vi "Decorator1_Main.vi"() -> ()   [LabVIEW 2020]
doc: "Main VI to test the DecoratorPattern"
uses:
  Espresso_class/Espresso.lvclass
  C:/Projects/DesignPatterns/DecoratorPattern/Beverage_class/Beverage.lvclass
  DarkRost_class/DarkRost.lvclass
  HouseBlend_class/HouseBlend.lvclass
  Decaf_class/Decaf.lvclass
  Milk_class/Milk.lvclass
  Soy_class/Soy.lvclass
  Mocha_class/Mocha.lvclass
  Whip_class/Whip.lvclass
  Beverage_class/Beverage.lvclass
panel:
  in  "Whip":u16(ring) items=["None", "Single", "Double"]
  in  "Mocha":u16(ring) items=["None", "Single", "Double"]
  in  "Coffee type":T1(radio)
  in  "Milk type":enum32{"No Milk", "Normal Milk", "Soy Milk"}(radio)
  out "Description and cost":string
  # "This Application shows how the Decorator Pattern could be implelemted based on the book:\nFirst Design Patterns,  Eric Freeman et. al. 2004. O'Reilly Media, Inc.\nhttp://oreilly.com/catalog/hfdesignpat/chapter/ch03.pdf\nCheers,\nMike"
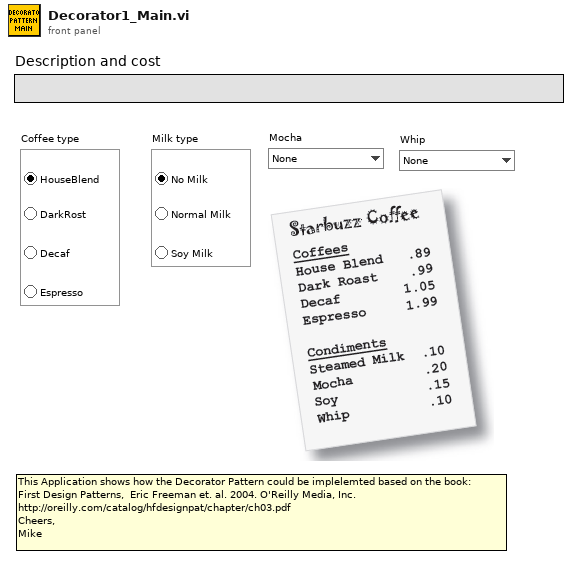
[diagram p1: front panel]
types:
  T1 = enum32{"HouseBlend", "DarkRost", "Decaf", "Espresso"}
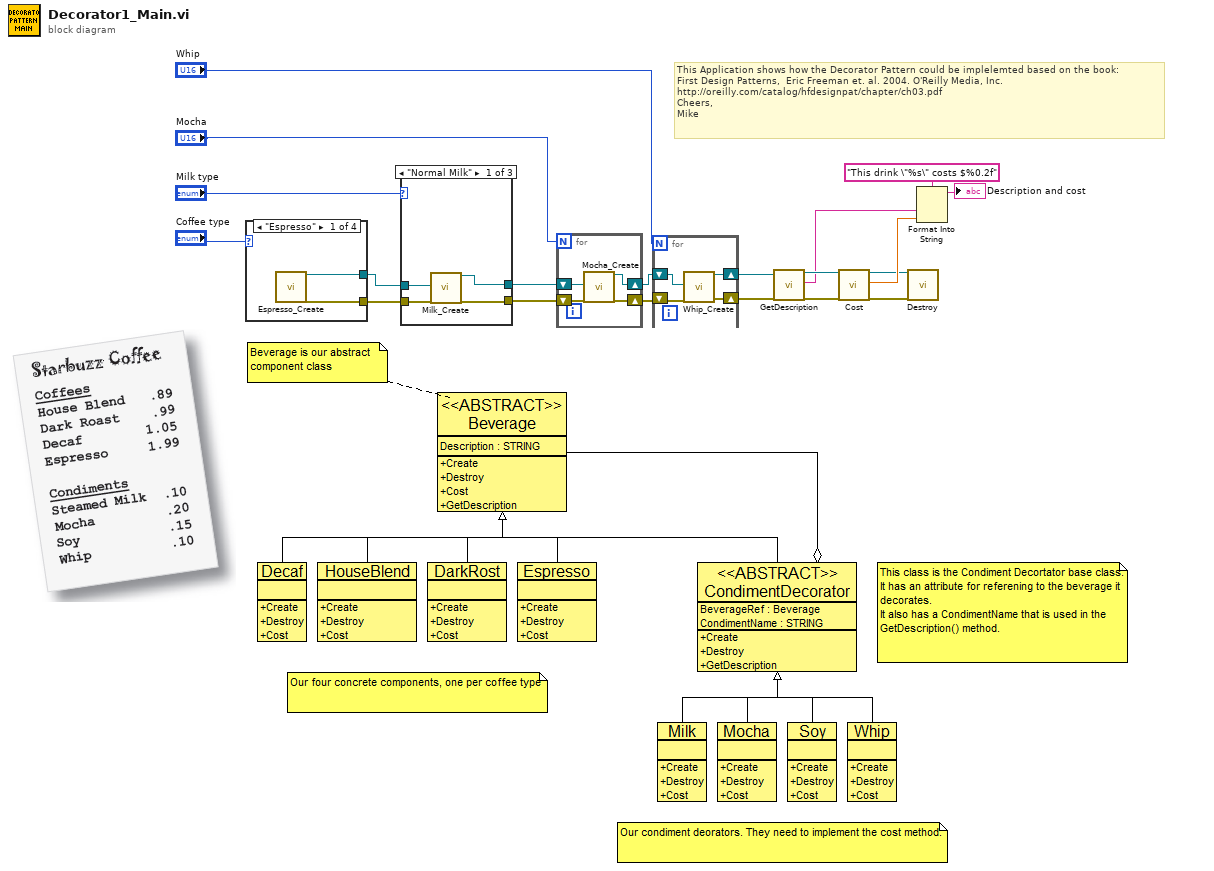
[diagram p0: block diagram]
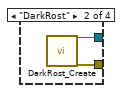
[diagram p2: hidden frame]
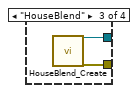
[diagram p3: hidden frame]
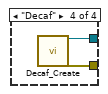
[diagram p4: hidden frame]
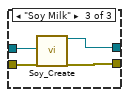
[diagram p6: hidden frame]
diagram:
  # "This Application shows how the Decorator Pattern could be implelemted based on the book:\nFirst Design Patterns,  Eric Freeman et. al. 2004. O'Reilly Media, Inc.\nhttp://oreilly.com/catalog/hfdesignpat/chapter/ch03.pdf\nCheers,\nMike"
  n1 = case shown="\"Espresso\"" "Coffee type" {
    tunnel: [w22 w24 w26 w28] -> w20
    tunnel: [w21 w23 w25 w27] -> w19
    frame "Espresso" {
      n2 = call "Espresso_Create.vi"() -> ("reference out"=w21:refnum<class "Espresso.lvclass">, "error out"=w22:errorcluster)  [unwired: 18 in]
    }
    frame "DarkRost" {
      n3 = call "DarkRost_Create.vi"() -> ("reference out"=w23:refnum<class "DarkRost.lvclass">, "error out"=w24:errorcluster)  [unwired: 18 in]
    }
    frame "HouseBlend" {
      n4 = call "HouseBlend_Create.vi"() -> ("reference out"=w25:refnum<class "HouseBlend.lvclass">, "error out"=w26:errorcluster)  [unwired: 18 in]
    }
    frame "Decaf" {
      n5 = call "Decaf_Create.vi"() -> ("reference out"=w27:refnum<class "Decaf.lvclass">, "error out"=w28:errorcluster)  [unwired: 18 in]
    }
  }
  n6 = case shown="\"Normal Milk\"" "Milk type" {
    tunnel: w20 -> [w32 w33 w38]
    tunnel: w19 -> [w31 w34 w35]
    tunnel: [w30 w33 w37] -> w18
    tunnel: [w29 w34 w36] -> w16
    frame "Normal Milk" {
      n7 = call "Milk_Create.vi"("Beverage"=w31, "error in (no error)"=w32) -> ("reference out"=w29:refnum<class "Milk.lvclass">, "error out"=w30:errorcluster)  [unwired: 16 in]
    }
    frame "No Milk" {
    }
    frame "Soy Milk" {
      n8 = call "Soy_Create.vi"("Beverage"=w35, "error in (no error)"=w38) -> ("reference out"=w36:refnum<class "Soy.lvclass">, "error out"=w37:errorcluster)  [unwired: 16 in]
    }
  }
  n9 = for {
    N: "Mocha" -> [_]
    shift-right: [w39] -> w15
    shift-left: w16 -> [w40]
    shift-right: [w41] -> w17
    shift-left: w18 -> [w42]
    n10 = call "Mocha_Create.vi"("Beverage"=w40, "error in (no error)"=w42) -> ("reference out"=w39:refnum<class "Mocha.lvclass">, "error out"=w41:errorcluster)  [unwired: 16 in]
  }
  n11 = for {
    N: "Whip" -> [_]
    shift-right: [w43] -> w2
    shift-left: w15 -> [w45]
    shift-right: [w44] -> w14
    shift-left: w17 -> [w46]
    n12 = call "Whip_Create.vi"("Beverage"=w45, "error in (no error)"=w46) -> ("reference out"=w43:refnum<class "Whip.lvclass">, "error out"=w44:errorcluster)  [unwired: 16 in]
  }
  n13 = call-dynamic "GetDescription.vi"("reference in"=w2, "error in (no error)"=w14) -> ("reference out"=w13:refnum<class "Beverage.lvclass">, "Description"=w6:string, "error out"=w12:errorcluster)  [unwired: 15 in]
  n14 = call-dynamic "Cost.vi"("reference in"=w13, "error in (no error)"=w12) -> ("reference out"=w9:refnum<class "Beverage.lvclass">, "Cost($)"=w10:dbl, "error out"=w8:errorcluster)  [unwired: 15 in]
  n15 = call-dynamic "Destroy.vi"("reference in"=w9, "error in (no error)"=w8) -> ()  [unwired: 16 in, 2 out]
  n16 = Format Into String(format string="This drink \"%s\" costs $%0.2f", w6, w10) -> (resulting string=→"Description and cost":string)  [unwired: 2 in, 1 out]
